vi "AlliGator Phasor Color Map User Event Refnum.vi"() -> (7 "Phasor Color Map Picker Event Refnum":refnum<user-event>)   [LabVIEW 2021, in "AlliGator Phasor Plot Color Map.lvlib"]
doc: "Stores the event refunm for the color map picker UI."
uses:
  AlliGator Phasor Plot Color Map.lvlib
  AlliGator Phasor Color Map User Event List.ctl
panel:
  # "see the AlliGator License on the block diagram (Ctrl+E or Window:Show Block Diagram)"
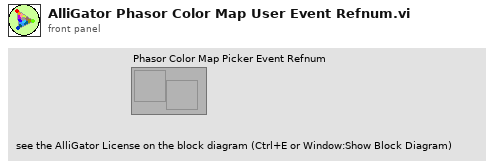
[diagram p1: front panel]
types:
  T1 = typedef "AlliGator Phasor Plot Color Map.lvlib/AlliGator Phasor Color Map User Event List.ctl" = enum16{"Init", "Vertex Update", "Color Change"}
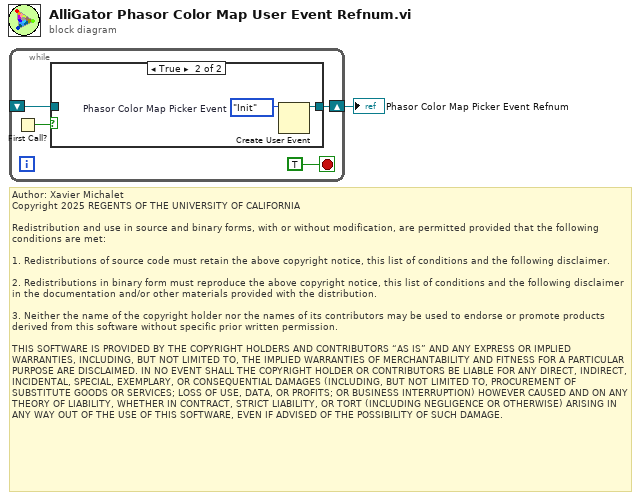
[diagram p0: block diagram]
diagram:
  # "Author: Xavier Michalet\nCopyright 2025 REGENTS OF THE UNIVERSITY OF CALIFORNIA\n\nRedistribution and use in source and binary forms, with or without modification, are permitted provided that the following conditions are met:\n\n1. Redistributions of source code must retain the above copyright notice, this list of conditions and the following disclaimer.\n\n2. Redistributions in binary form must reproduce the above copyright notice, this list of conditions and the following disclaimer in the documentation and/or other materials provided with the distribution.\n\n3. Neither the name of the copyright holder nor the names of its contributors may be used to endorse or promote products derived from this software without specific prior written permission.\n\nTHIS SOFTWARE IS PROVIDED BY THE COPYRIGHT HOLDERS AND CONTRIBUTORS “AS IS” AND ANY EXPRESS OR IMPLIED WARRANTIES, INCLUDING, BUT NOT LIMITED TO, THE IMPLIED WARRANTIES OF MERCHANTABILITY AND FITNESS FOR A PARTICULAR PURPOSE ARE DISCLAIMED. IN NO EVENT SHALL THE COPYRIGHT HOLDER OR CONTRIBUTORS BE LIABLE FOR ANY DIRECT, INDIRECT, INCIDENTAL, SPECIAL, EXEMPLARY, OR CONSEQUENTIAL DAMAGES (INCLUDING, BUT NOT LIMITED TO, PROCUREMENT OF SUBSTITUTE GOODS OR SERVICES; LOSS OF USE, DATA, OR PROFITS; OR BUSINESS INTERRUPTION) HOWEVER CAUSED AND ON ANY THEORY OF LIABILITY, WHETHER IN CONTRACT, STRICT LIABILITY, OR TORT (INCLUDING NEGLIGENCE OR OTHERWISE) ARISING IN ANY WAY OUT OF THE USE OF THIS SOFTWARE, EVEN IF ADVISED OF THE POSSIBILITY OF SUCH DAMAGE."
  n1 = while {
    shift-right: [w3] -> w1
    shift-left: _ -> [w2]
    stop <- TRUE stop-if-true
    n2 = First Call?() -> (First Call?: T/F=w4:bool)
    n3 = case shown="True" w4 {
      tunnel: [w6 w7] -> w3
      tunnel: w2 -> [w6 _]
      frame False {
      }
      frame True {
        w8 = AlliGator_Phasor_Color_Map_User_Event_List."Init"  # Phasor Color Map Picker Event
        n4 = Create User Event(user event datatype=w8) -> (user event=w7:refnum<user-event>)  [unwired: 1 in, 1 out]
      }
    }
  }
  "Phasor Color Map Picker Event Refnum" <- w1
